vi "Calc_Extention_ver2.vi"(8 "Center State at T":T2, 9 "Initial Anchor Position":dbl[][](array[numeric]), 11 "On_Particle State":T1(array[cluster])) -> (0 "New Center State at T":T2, 2 "Extension":dbl[][](array[numeric]), 3 "On_Particle State":T1(array[cluster]))   [LabVIEW 2020]
uses:
  <vilib>/Analysis/baseanly.llb/Mean (DBL).vi
  <vilib>/Analysis/NI_AALBase.lvlib
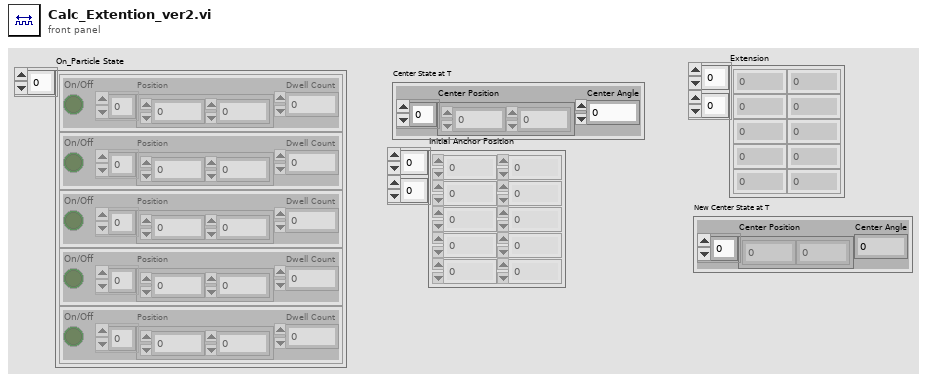
[diagram p1: front panel]
types:
  T1 = cluster{"On/Off":bool, "Position":dbl[], "Dwell Count":i32}[]
  T2 = cluster{"Center Position":dbl[], "Center Angle":dbl}
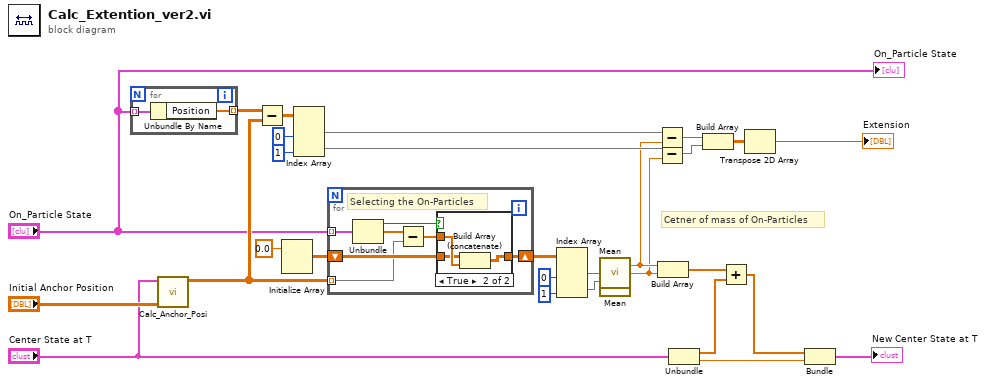
[diagram p0: block diagram]
diagram:
  # "Cetner of mass of On-Particles"
  n1 = for {
    tunnel: "On_Particle State" -> [w30] mode=indexing
    tunnel: [w29] -> w13 mode=indexing
    n2 = Unbundle By Name(w30) -> ("Position"=w29:dbl[])
  }
  n3 = call "Calc_Anchor_Posi.vi"("Initial Anchor Position"="Initial Anchor Position", "Center State at T"="Center State at T") -> ("Anchor Posi at T"=w5:dbl[][])  [unwired: 9 in]
  n4 = Subtract(x=w13, y=w5) -> (x-y=w19:dbl[][])
  n5 = Initialize Array(0.0 ("element")) -> (w11:dbl[][])  [unwired: 2 in]
  n6 = Index Array(array=w19, index (col) #1=0 ("disabled index (col)"), index (col) #2=1 ("index (col)")) -> (element #1=w26:dbl[], element #2=w25:dbl[])  [unwired: 2 in]
  n7 = for {
    tunnel: "On_Particle State" -> [w37] mode=indexing
    shift-right: [w34] -> w10
    shift-left: w11 -> [w35]
    tunnel: w5 -> [w32] mode=indexing
    # "Selecting the On-Particles"
    n8 = Unbundle(w37) -> ("On/Off"=w36:bool, "Position"=w33:dbl[])  [unwired: 1 out]
    n9 = Subtract(x=w33, y=w32) -> (x-y=w31:dbl[])
    n10 = case shown="TRUE" w36 {
      tunnel: w31 -> [_ w41]
      tunnel: w35 -> [w38 w40]
      tunnel: [w38 w39] -> w34
      frame False {
      }
      frame True {
        n11 = Build Array (concatenate)(w40, w41) -> (w39:dbl[][])
      }
    }
  }
  n12 = Index Array(array=w10, index (col) #1=0 ("disabled index (col)"), index (col) #2=1 ("index (col)")) -> (element #1=w7:dbl[], element #2=w6:dbl[])  [unwired: 2 in]
  n13 = call-poly <vilib>:"Mean.vi"("X"=w7) -> ("mean"=w21:dbl)  [unwired: 1 out]
  n14 = call-poly <vilib>:"Mean.vi"("X"=w6) -> ("mean"=w20:dbl)  [unwired: 1 out]
  n15 = Subtract(x=w26, y=w21) -> (x-y=w24:dbl[])
  n16 = Subtract(x=w25, y=w20) -> (x-y=w23:dbl[])
  n17 = Build Array(w21, w20) -> (w3:dbl[])
  n18 = Unbundle("Center State at T") -> ("Center Position"=w2:dbl[], "Center Angle"=w15:dbl)
  n19 = Build Array(w24, w23) -> (w22:dbl[][])
  n20 = Add(x=w3, y=w2) -> (x+y=w1:dbl[])
  n21 = Transpose 2D Array(2D array=w22) -> (transposed array=→"Extension":dbl[][])
  n22 = Bundle(w1, "Center Angle"=w15) -> (→"New Center State at T":cluster{dbl[], "Center Angle":dbl})  [unwired: 1 in]
  "On_Particle State" <- "On_Particle State"
